vi "Reset.vi"(0 "Display State In":T1, 9 "Container State":T4, 11 "error in (no error)":errorcluster) -> (4 "Display State Out":T1, 15 "error out":errorcluster)   [LabVIEW 2011, in "VariantXControl__VP.xctl"]
uses:
  VariantXControl__VP.xctl
  <vilib>/_xctls/Container State.ctl
  VariantState.ctl
  Permissions.ctl
  TreeSettings.ctl
  <vilib>/_xctls/XControlSupport.lvlib
types:
  T1 = typedef "VariantXControl__VP.xctl/VariantState.ctl" = cluster{"State":string, "Messages":cluster{"Message":string, "Parameter":variant}[], "Current run":i32, "Start run":i32, "LastTag":string, "Tags":string[], "Length":i32, "Permissions":T2, "IsProbe?":bool, "Changed":bool, "TreeSettings":T3, "Tree Ref":refnum<vi>}
  T2 = typedef "VariantXControl__VP.xctl/Permissions.ctl" = cluster{"Reset":bool, "TraverseAttributes":bool, "Colorize":bool}
  T3 = typedef "VariantXControl__VP.xctl/TreeSettings.ctl" = cluster{"Traverse":bool, "Colorize":bool}
  T4 = typedef "XControlSupport.lvlib/Container State.ctl" = cluster{"Indicator?":bool, "Run Mode?":bool, " Refnum":refnum<vi>}
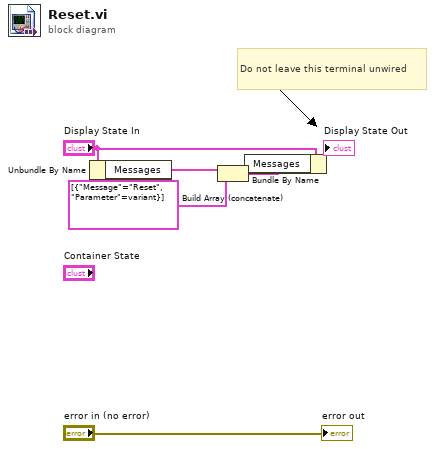
[diagram p0: block diagram]
diagram:
  # "Do not leave this terminal unwired"
  n1 = Unbundle By Name("Display State In") -> ("Messages"=w3:cluster{"Message":string, "Parameter":variant}[])
  n2 = Build Array (concatenate)(w3, cluster{"Message":string, "Parameter":variant}[] [{"Message"="Reset", "Parameter"=variant}] ("array")) -> (w2:cluster{"Message":string, "Parameter":variant}[])
  n3 = Bundle By Name(cluster="Display State In", "Messages"=w2) -> (→"Display State Out":T1)
  "error out" <- "error in (no error)"
